vi "Send Message.vi"(6 "Message Priority":enum16{"Normal", "High"}(ring), 8 "error in":errorcluster, 10 "Message Payload in":refnum<class "IMessagePayload.lvclass">, 11 "NotifierMessageTransport in":refnum<class "NotifierMessageTransport.lvclass">) -> (0 "error out":errorcluster, 3 "NotifierMessageTransport out":refnum<class "NotifierMessageTransport.lvclass">)   [LabVIEW 2016, in "NotifierMessageTransport.lvclass"]
uses:
  NotifierMessageTransport.lvclass
  IMessagePayload/IMessagePayload.lvclass
panel:
  # "INPUTS"
  # "OUTPUTS"
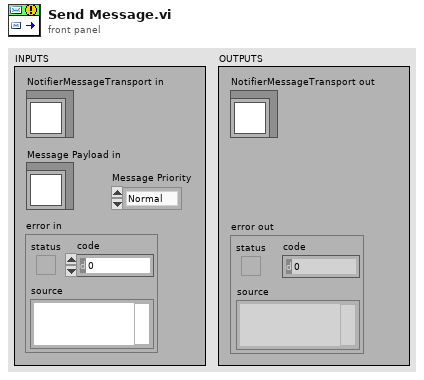
[diagram p1: front panel]
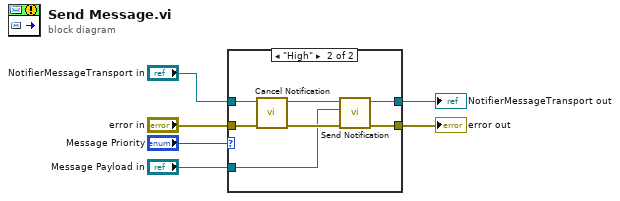
[diagram p0: block diagram]
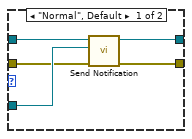
[diagram p2: hidden frame]
diagram:
  n1 = case shown="\"High\"" "Message Priority" {
    tunnel: "NotifierMessageTransport in" -> [w11 w18]
    tunnel: "Message Payload in" -> [w10 w14]
    tunnel: "error in" -> [w9 w17]
    tunnel: [w8 w12] -> w3
    tunnel: [w7 w13] -> w2
    frame "Normal", Default {
      n2 = call "Send Notification.vi"("error in"=w9, "IMessagePayload.lvclass"=w10, "NotifierMessageTransport in"=w11) -> ("error out"=w7:errorcluster, "NotifierMessageTransport out"=w8:refnum<class "NotifierMessageTransport.lvclass">)  [unwired: 7 in]
    }
    frame "High" {
      n3 = call "Cancel Notification.vi"("error in"=w17, "NotifierMessageTransport in"=w18) -> ("error out"=w16:errorcluster, "NotifierMessageTransport out"=w15:refnum<class "NotifierMessageTransport.lvclass">)  [unwired: 8 in]
      n4 = call "Send Notification.vi"("error in"=w16, "IMessagePayload.lvclass"=w14, "NotifierMessageTransport in"=w15) -> ("error out"=w13:errorcluster, "NotifierMessageTransport out"=w12:refnum<class "NotifierMessageTransport.lvclass">)  [unwired: 7 in]
    }
  }
  "error out" <- w2
  "NotifierMessageTransport out" <- w3
